vi "ADI_IMU_ADIS16470_FGV.vi"(0 "ADI IMU DevRef":T2={"DevStatus"={"status"=FALSE, "code"=0, "source"=""}, "Handle"=0, "SPI Bus"=enum."SPI On-Board, CS0", "Device Found"=FALSE, "Device Ready"=FALSE, "Yaw Axis"=enum."Z", "Serial"=0, "Bytes Per Sample"=0, "Calibrate On Open?"=FALSE}, 1 "Operation":enum16{"set", "get", "set reset"}(ring), 2 "Sensor Ready?":bool, 5 "Reset":bool, 7 "IMU Data":T1, 9 "IMU Angles":T4, 12 "Offset Compensated Data":dbl[](array[numeric])) -> (4 "ADI IMU DevRef Out":T2={"DevStatus"={"status"=FALSE, "code"=0, "source"=""}, "Handle"=0, "SPI Bus"=enum."SPI On-Board, CS0", "Device Found"=FALSE, "Device Ready"=FALSE, "Yaw Axis"=enum."Z", "Serial"=0, "Bytes Per Sample"=0, "Calibrate On Open?"=FALSE}, 6 "Reset Out":bool, 8 "IMU Data":T1, 10 "IMU Angles Out":T4, 13 "Sensor Ready Out":bool, 14 "Offset Compensated Data Out":dbl[](array[numeric]))   [LabVIEW 2017, in "ADIS16470_IMU.lvlib"]
uses:
  ADIS16470_IMU.lvlib
  ADI_IMU_ADIS16470_IMUDevRef.ctl
  <vilib>/Rock Robotics/SystemInterfaces/spilib/spi_bus.ctl
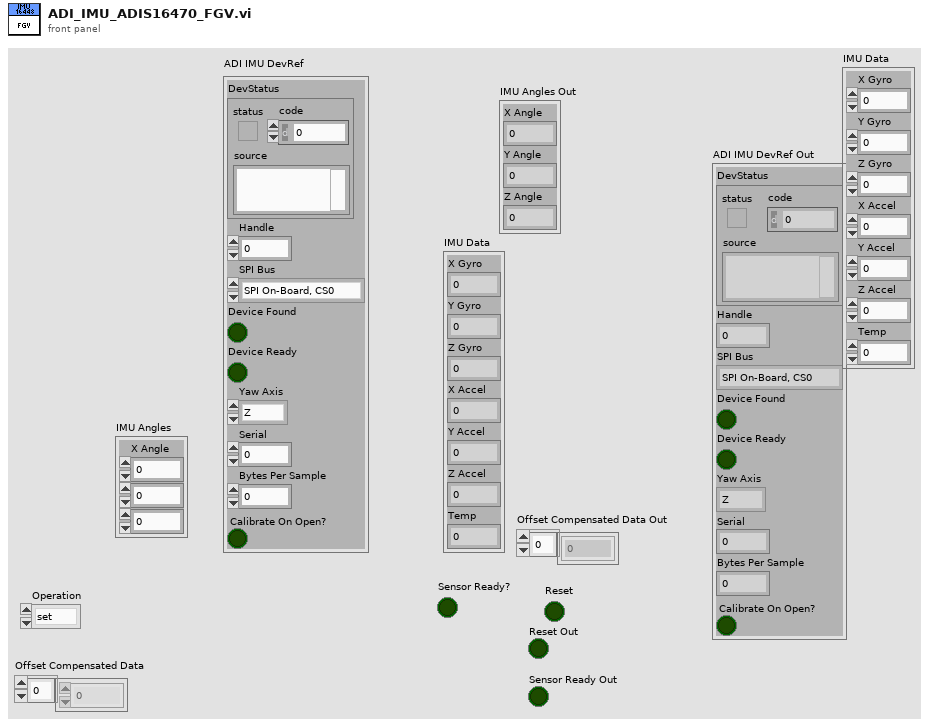
[diagram p1: front panel]
types:
  T1 = cluster{"X Gyro":dbl, "Y Gyro":dbl, "Z Gyro":dbl, "X Accel":dbl, "Y Accel":dbl, "Z Accel":dbl, "Temp":dbl}
  T2 = typedef "ADIS16470_IMU.lvlib/ADI_IMU_ADIS16470_IMUDevRef.ctl" = cluster{"DevStatus":errorcluster, "Handle":i32, "SPI Bus":T3, "Device Found":bool, "Device Ready":bool, "Yaw Axis":enum16{"X", "Y", "Z"}, "Serial":u16, "Bytes Per Sample":u16, "Calibrate On Open?":bool}
  T3 = typedef "spi_bus.ctl" = enum16{"SPI On-Board, CS0", "SPI On-Board, CS1", "SPI On-Board, CS2", "SPI On-Board, CS3", "SPI MXP", "Invalid"}
  T4 = cluster{"X Angle":dbl, "Y Angle":dbl, "Z Angle":dbl}
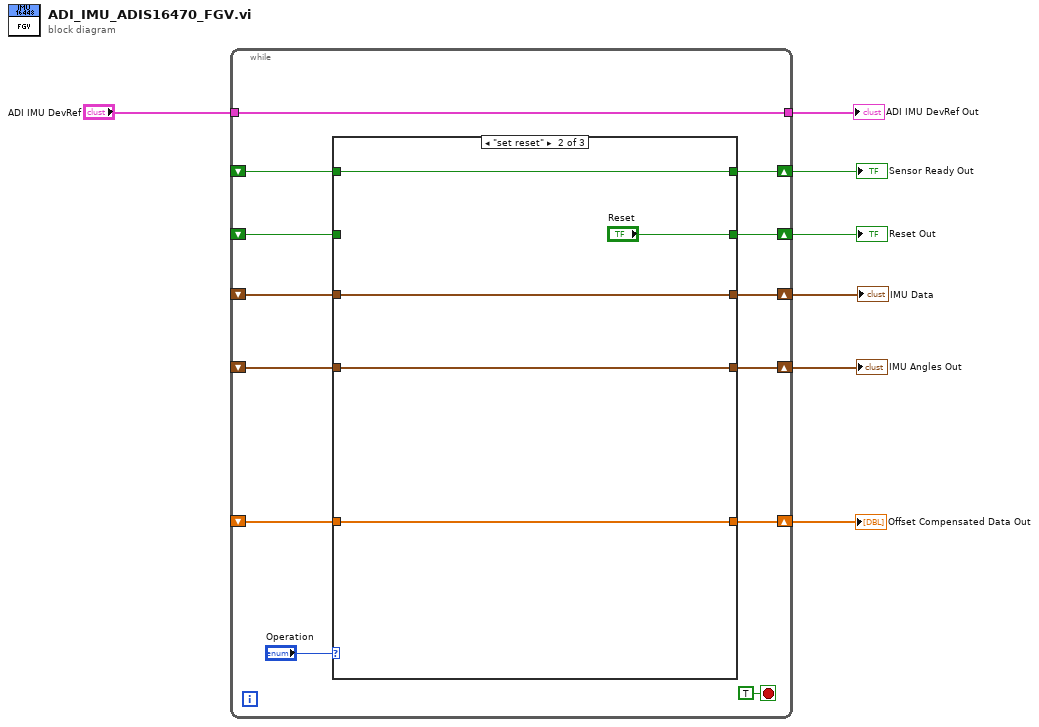
[diagram p0: block diagram]
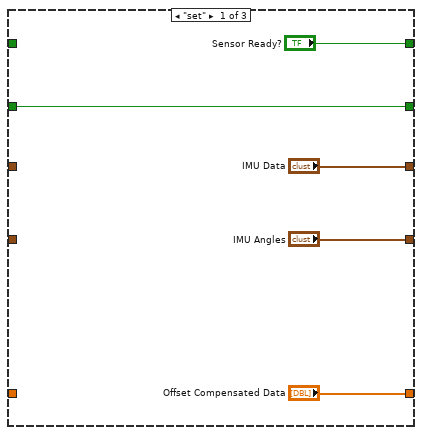
[diagram p2: hidden frame]
diagram:
  n1 = while {
    shift-right: [w18] -> w7
    shift-left: _ -> [w12]
    shift-right: [w17] -> w4
    shift-left: _ -> [w13]
    tunnel: "ADI IMU DevRef" -> [w16]
    tunnel: [w16] -> w5
    shift-right: [w15] -> w3
    shift-left: _ -> [w14]
    shift-right: [w11] -> w1
    shift-left: _ -> [w10]
    shift-right: [w8] -> w6
    shift-left: _ -> [w9]
    stop <- TRUE stop-if-true
    n2 = case shown="\"set reset\"" "Operation" {
      tunnel: [w23 "Reset" w33] -> w18
      tunnel: ["IMU Data" w27 w34] -> w17
      tunnel: ["IMU Angles" w28 w35] -> w15
      tunnel: w14 -> [_ w28 w35]
      tunnel: w13 -> [_ w27 w34]
      tunnel: w12 -> [w23 _ w33]
      tunnel: ["Offset Compensated Data" w29 w32] -> w11
      tunnel: w10 -> [_ w29 w32]
      tunnel: ["Sensor Ready?" w26 w31] -> w8
      tunnel: w9 -> [_ w26 w31]
      frame "set" {
      }
      frame "set reset" {
      }
      frame "get", Default {
      }
    }
  }
  "Reset Out" <- w7
  "Sensor Ready Out" <- w6
  "IMU Angles Out" <- w3
  "ADI IMU DevRef Out" <- w5
  "Offset Compensated Data Out" <- w1
  "IMU Data" <- w4
